vi "Load Config.vi"(11 "configuration file path":path=path "C:/Users/telsey/Desktop/Personal Projects/Photobooth/Photobooth.ini") -> (0 "Images":path, 1 "Header":path, 2 "Photoset":string, 3 "Flickr Enabled":bool, 5 "Photoset Description":string)   [LabVIEW 2010]
uses:
  <vilib>/Utility/config.llb/Read Key (Boolean).vi
  <vilib>/Utility/config.llb/Read Key (String).vi
  <vilib>/Utility/config.llb/Read Key (Path).vi
  <vilib>/Utility/config.llb/NI_LVConfig.lvlib
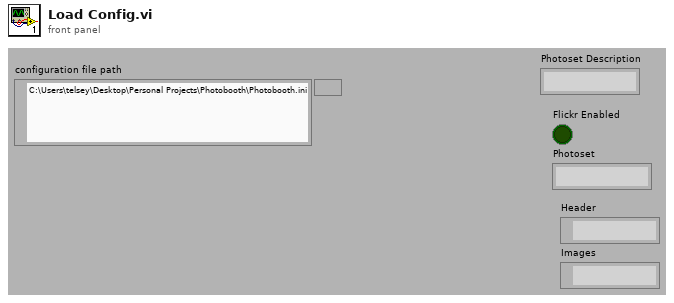
[diagram p1: front panel]
types:
  T1 = typedef "NI_LVConfig.lvlib/Config Data RefNum.ctl" = refnum<k1>
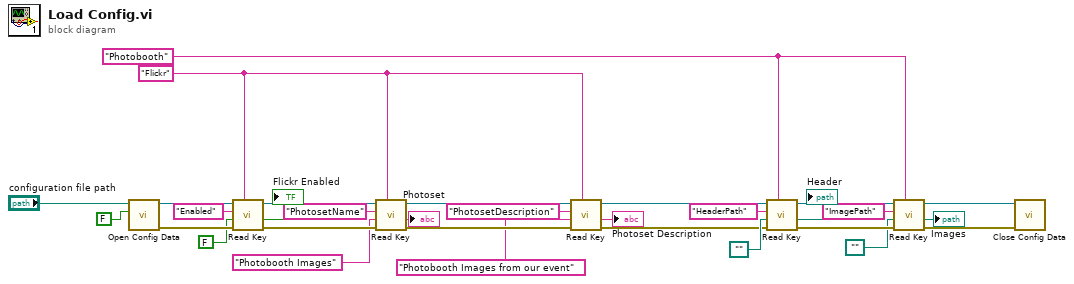
[diagram p0: block diagram]
diagram:
  w23 = "Photobooth" ("section")
  w1 = "Flickr" ("section")
  n1 = call <vilib>:"Open Config Data.vi"("create file if necessary (T)"=FALSE, "configuration file path"="configuration file path") -> ("error out"=w24:errorcluster, "refnum"=w31:T1)  [unwired: 7 in, 1 out]
  n2 = call-poly <vilib>:"Read Key.vi"("section"=w1, "error in (no error)"=w24, "default value"=FALSE, "key"="Enabled", "refnum"=w31) -> ("error out"=w22:errorcluster, "value"=→"Flickr Enabled":bool, "refnum out"=w30:T1)  [unwired: 3 in, 1 out]
  n3 = call-poly <vilib>:"Read Key.vi"("section"=w1, "error in (no error)"=w22, "default value"="Photobooth Images", "key"="PhotosetName", "refnum"=w30) -> ("error out"=w5:errorcluster, "value"=→"Photoset":string, "refnum out"=w29:T1)  [unwired: 3 in, 1 out]
  n4 = call-poly <vilib>:"Read Key.vi"("section"=w1, "error in (no error)"=w5, "default value"="Photobooth Images from our event", "key"="PhotosetDescription", "refnum"=w29) -> ("error out"=w6:errorcluster, "value"=→"Photoset Description":string, "refnum out"=w7:T1)  [unwired: 3 in, 1 out]
  n5 = call-poly <vilib>:"Read Key.vi"("section"=w23, "error in (no error)"=w6, "default value"=path "", "key"="HeaderPath", "refnum"=w7) -> ("error out"=w21:errorcluster, "value"=→"Header":path, "refnum out"=w28:T1)  [unwired: 3 in, 1 out]
  n6 = call-poly <vilib>:"Read Key.vi"("section"=w23, "error in (no error)"=w21, "default value"=path "", "key"="ImagePath", "refnum"=w28) -> ("error out"=w20:errorcluster, "value"=→"Images":path, "refnum out"=w27:T1)  [unwired: 3 in, 1 out]
  n7 = call <vilib>:"Close Config Data.vi"("error in (no error)"=w20, "refnum"=w27) -> ()  [unwired: 8 in, 2 out]
